vi "Set Buffer Offset.vi"(10 "buffer offset":u64 format="%d bytes", 11 "Buffer in":refnum<class "Buffer.lvclass">) -> (3 "Buffer out":refnum<class "Buffer.lvclass">)   [LabVIEW 2017, in "DSF Core.lvlib" / "Buffer.lvclass"]
uses:
  Buffer.lvclass
  Buffer.lvclass/Buffer.ctl
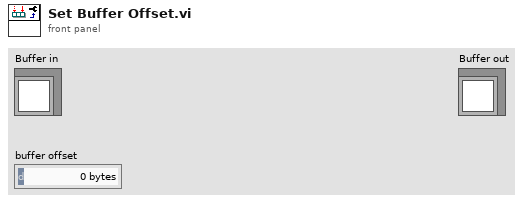
[diagram p1: front panel]
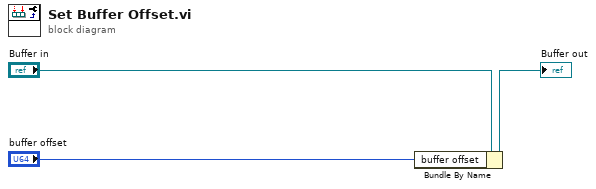
[diagram p0: block diagram]
diagram:
  n1 = Bundle By Name(cluster="Buffer in", "buffer offset"="buffer offset") -> (→"Buffer out":refnum<class "Buffer.lvclass">)
